vi "LargeNetworks.vi"() -> ()   [LabVIEW 2022 SP3]
uses:
  MOTION/TypeDefs/EL72xx_DMCOutputs.ctl
  MOTION/TypeDefs/EL72xx_DMCInputs.ctl
  SAFETY/TypeDefs/TwinSAFEGroupInfoData.ctl
  SAFETY/TypeDefs/FSLogicInputs.ctl
  SAFETY/TypeDefs/DeviceInfoData.ctl
  IO/TypeDefs/EL2008Outputs.ctl
  SAFETY/TypeDefs/TwinSAFETerminal.ctl
  <userlib>/Beckhoff-LabVIEW-Interface/Utilities/Notification/Buffered User-Event Data.ctl
  <userlib>/Beckhoff-LabVIEW-Interface/_DependsOn/Base/Read/Register E-Notification Buffered.vi
  <userlib>/Beckhoff-LabVIEW-Interface/_DependsOn/Base/Read/Read Sync.vi
  <userlib>/Beckhoff-LabVIEW-Interface/_DependsOn/Base/TypeResolver/Get TypeResolver.vi
  MOTION/Motion_Library.lvlib
  ADS/ADS_Library.lvlib
  SAFETY/Safety_Library.lvlib
  IO/IO_Library.lvlib
panel:
  out "bHasMatched 3":bool
  out "Write Status 3":bool
  in  "NI9472":T1
  in  "Digital Outputs 2":string="<PortInfo><Inputs><SymbolControlItems><SymbolControlItem GroupName=\"ADS Write\" GroupDescription=\"Parameters for ADS Write command\"><Parameters><Parameter Name=\"Name\">Box 17 (NI 9145).Module 1 (NI 9472).Digital Output.DO</Parameter><Parameter Name=\"SymbolName\">Box 17 (NI 9145).Module 1 (NI 9472).Digital Output.DO</Parameter><Parameter Name=\"SymbolType\">USINT</Parameter><Parameter Name=\"SymbolGuid\"></Parameter><Parameter Name=\"AmsNetId\">10.97.0.23.1.1</Parameter><Parameter Name=\"Port\">27911</Parameter><Parameter Name=\"IndexGroup\">#x0</Parameter><Parameter Name=\"IndexOffset\">#x0</Parameter><Parameter Name=\"BitSize\">8</Parameter><Parameter Name=\"CycleTime [ms]\">10</Parameter><Parameter Name=\"Timeout [ms]\">1000</Parameter></Parameters></SymbolControlItem></SymbolControlItems></Inputs><Outputs><SymbolControlItems /></Outputs></PortInfo>"
  out "error out 5":errorcluster
  in  "error in (no error) 2":errorcluster
  out "EL2904":T2
  out "EL1904":T2
  in  "stop":bool
  out "Read status? 3":bool
  out "RDataArray":variant[](array[variant])
  out "RData":variant
  out "Waveform Chart 2":dbl(graph)
  out "error out 4":errorcluster
  in  "error in 2":errorcluster
  in  "String":string="<PortInfo><Inputs><SymbolControlItems /></Inputs><Outputs><SymbolControlItems><SymbolControlItem GroupName=\"ADS Read\" GroupDescription=\"Parameters for ADS Read command\"><Parameters><Parameter Name=\"Name\">Term 15 (EL3255).AI Standard Channel 1.Value</Parameter><Parameter Name=\"SymbolName\">Term 15 (EL3255).AI Standard Channel 1.Value</Parameter><Parameter Name=\"SymbolType\">INT</Parameter><Parameter Name=\"SymbolGuid\"></Parameter><Parameter Name=\"AmsNetId\">10.97.0.23.1.1</Parameter><Parameter Name=\"Port\">27911</Parameter><Parameter Name=\"IndexGroup\">#x0</Parameter><Parameter Name=\"IndexOffset\">#x0</Parameter><Parameter Name=\"BitSize\">16</Parameter><Parameter Name=\"CycleTime [ms]\">10</Parameter><Parameter Name=\"Transmode\">3</Parameter><Parameter Name=\"Timeout [ms]\">1000</Parameter><Parameter Name=\"TCBufferSize [Samples]\">10</Parameter><Parameter Name=\"LVBufferSize [Samples]\">50</Parameter><Parameter Name=\"Expected min delay [ms]\">500</Parameter></Parameters></SymbolControlItem></SymbolControlItems></Outputs></PortInfo>"
  in  "Digital Outputs":string="<PortInfo><Inputs><SymbolControlItems><SymbolControlItem GroupName=\"ADS Write\" GroupDescription=\"Parameters for ADS Write command\"><Parameters><Parameter Name=\"Name\">Term 2 (EL2008).Channel 1.Output</Parameter><Parameter Name=\"SymbolName\">Term 2 (EL2008).Channel 1.Output</Parameter><Parameter Name=\"SymbolType\">BIT</Parameter><Parameter Name=\"SymbolGuid\"></Parameter><Parameter Name=\"AmsNetId\">10.97.0.23.1.1</Parameter><Parameter Name=\"Port\">27905</Parameter><Parameter Name=\"IndexGroup\">#x0</Parameter><Parameter Name=\"IndexOffset\">#x0</Parameter><Parameter Name=\"BitSize\">1</Parameter><Parameter Name=\"CycleTime [ms]\">2</Parameter><Parameter Name=\"Timeout [ms]\">1000</Parameter></Parameters></SymbolControlItem><SymbolControlItem GroupName=\"ADS Write\" GroupDescription=\"Parameters for ADS Write command\"><Parameters><Parameter Name=\"Name\">Term 2 (EL2008).Channel 2.Output</Parameter><Parameter Name=\"SymbolName\">Term 2 (EL2008).Channel 2.Output</Parameter><Parameter Name=\"SymbolType\">BIT</Parameter><Parameter Name=\"SymbolGuid\"></Parameter><Parameter Name=\"AmsNetId\">10.97.0.23.1.1</Parameter><Parameter Name=\"Port\">27905</Parameter><Parameter Name=\"IndexGroup\">#x0</Parameter><Parameter Name=\"IndexOffset\">#x0</Parameter><Parameter Name=\"BitSize\">1</Parameter><Parameter Name=\"CycleTime [ms]\">2</Parameter><Parameter Name=\"Timeout [ms]\">1000</Parameter></Parameters></SymbolControlItem><SymbolControlItem GroupName=\"ADS Write\" GroupDescription=\"Parameters for ADS Write command\"><Parameters><Parameter Name=\"Name\">Term 2 (EL2008).Channel 3.Output</Parameter><Parameter Name=\"SymbolName\">Term 2 (EL2008).Channel 3.Output</Parameter><Parameter Name=\"SymbolType\">BIT</Parameter><Parameter Name=\"SymbolGuid\"></Parameter><Parameter Name=\"AmsNetId\">10.97.0.23.1.1</Parameter><Parameter Name=\"Port\">27905</Parameter><Parameter Name=\"IndexGroup\">#x0</Parameter><Parameter Name=\"IndexOffset\">#x0</Parameter><Parameter Name=\"BitSize\">1</Parameter><Parameter Name=\"CycleTime [ms]\">2</Parameter><Parameter Name=\"Timeout [ms]\">1000</Parameter></Parameters></SymbolControlItem><SymbolControlItem GroupName=\"ADS Write\" GroupDescription=\"Parameters for ADS Write command\"><Parameters><Parameter Name=\"Name\">Term 2 (EL2008).Channel 4.Output</Parameter><Parameter Name=\"SymbolName\">Term 2 (EL2008).Channel 4.Output</Parameter><Parameter Name=\"SymbolType\">BIT</Parameter><Parameter Name=\"SymbolGuid\"></Parameter><Parameter Name=\"AmsNetId\">10.97.0.23.1.1</Parameter><Parameter Name=\"Port\">27905</Parameter><Parameter Name=\"IndexGroup\">#x0</Parameter><Parameter Name=\"IndexOffset\">#x0</Parameter><Parameter Name=\"BitSize\">1</Parameter><Parameter Name=\"CycleTime [ms]\">2</Parameter><Parameter Name=\"Timeout [ms]\">1000</Parameter></Parameters></SymbolControlItem><SymbolControlItem GroupName=\"ADS Write\" GroupDescription=\"Parameters for ADS Write command\"><Parameters><Parameter Name=\"Name\">Term 2 (EL2008).Channel 5.Output</Parameter><Parameter Name=\"SymbolName\">Term 2 (EL2008).Channel 5.Output</Parameter><Parameter Name=\"SymbolType\">BIT</Parameter><Parameter Name=\"SymbolGuid\"></Parameter><Parameter Name=\"AmsNetId\">10.97.0.23.1.1</Parameter><Parameter Name=\"Port\">27905</Parameter><Parameter Name=\"IndexGroup\">#x0</Parameter><Parameter Name=\"IndexOffset\">#x0</Parameter><Parameter Name=\"BitSize\">1</Parameter><Parameter Name=\"CycleTime [ms]\">2</Parameter><Parameter Name=\"Timeout [ms]\">1000</Parameter></Parameters></SymbolControlItem><SymbolControlItem GroupName=\"ADS Write\" GroupDescription=\"Parameters for ADS Write command\"><Parameters><Parameter Name=\"Name\">Term 2 (EL2008).Channel 6.Output</Parameter><Parameter Name=\"SymbolName\">Term 2 (EL2008).Channel 6.Output</Parameter><Parameter Name=\"SymbolType\">BIT</Parameter><Parameter Name=\"SymbolGuid\"></Parameter><Parameter Name=\"AmsNetId\">10.97.0.23.1.1</Parameter><Parameter Name=\"Port\">27905</Parameter><Parameter Name=\"IndexGroup\">#x0</Parameter><Parameter Name=\"IndexOffset\">#x0</Parameter><Parameter Name=\"BitSize\">1</Parameter><Parameter Name=\"CycleTime [ms]\">2</Parameter><Parameter Name=\"Timeout [ms]\">1000</Parameter></Parameters></SymbolControlItem><SymbolControlItem GroupName=\"ADS Write\" GroupDescription=\"Parameters for ADS Write command\"><Parameters><Parameter Name=\"Name\">Term 2 (EL2008).Channel 7.Output</Parameter><Parameter Name=\"SymbolName\">Term 2 (EL2008).Channel 7.Output</Parameter><Parameter Name=\"SymbolType\">BIT</Parameter><Parameter Name=\"SymbolGuid\"></Parameter><Parameter Name=\"AmsNetId\">10.97.0.23.1.1</Parameter><Parameter Name=\"Port\">27905</Parameter><Parameter Name=\"IndexGroup\">#x0</Parameter><Parameter Name=\"IndexOffset\">#x0</Parameter><Parameter Name=\"BitSize\">1</Parameter><Parameter Name=\"CycleTime [ms]\">2</Parameter><Parameter Name=\"Timeout [ms]\">1000</Parameter></Parameters></SymbolControlItem><SymbolControlItem GroupName=\"ADS Write\" GroupDescription=\"Parameters for ADS Write command\"><Parameters><Parameter Name=\"Name\">Term 2 (EL2008).Channel 8.Output</Parameter><Parameter Name=\"SymbolName\">Term 2 (EL2008).Channel 8.Output</Parameter><Parameter Name=\"SymbolType\">BIT</Parameter><Parameter Name=\"SymbolGuid\"></Parameter><Parameter Name=\"AmsNetId\">10.97.0.23.1.1</Parameter><Parameter Name=\"Port\">27905</Parameter><Parameter Name=\"IndexGroup\">#x0</Parameter><Parameter Name=\"IndexOffset\">#x0</Parameter><Parameter Name=\"BitSize\">1</Parameter><Parameter Name=\"CycleTime [ms]\">2</Parameter><Parameter Name=\"Timeout [ms]\">1000</Parameter></Parameters></SymbolControlItem></SymbolControlItems></Inputs><Outputs><SymbolControlItems /></Outputs></PortInfo>"
  out "error out 3":errorcluster
  out "Write Status 2":bool[](array[boolean])
  out "bHasMatched 2":bool[](array[boolean])
  in  "EL2008 Channels":T1
  in  "error in (no error)":errorcluster
  out "SymbolName":string
  in  "Start Notifications":bool=TRUE
  out "Waveform Chart":sgl(graph)
  in  "Stop Notifications":bool
  out "Has stopped?":bool
  out "Has started?":bool
  out "error out 2":errorcluster
  in  "error in":errorcluster
  in  "Counter":string="<PortInfo><Inputs><SymbolControlItems /></Inputs><Outputs><SymbolControlItems><SymbolControlItem GroupName=\"ADS Read\" GroupDescription=\"Parameters for ADS Read command\"><Parameters><Parameter Name=\"Name\">Term 14 (EL5021-0090).ENC Status.Counter value</Parameter><Parameter Name=\"SymbolName\">Term 14 (EL5021-0090).ENC Status.Counter value</Parameter><Parameter Name=\"SymbolType\">UDINT</Parameter><Parameter Name=\"SymbolGuid\"></Parameter><Parameter Name=\"AmsNetId\">10.97.0.23.1.1</Parameter><Parameter Name=\"Port\">27911</Parameter><Parameter Name=\"IndexGroup\">#x0</Parameter><Parameter Name=\"IndexOffset\">#x0</Parameter><Parameter Name=\"BitSize\">32</Parameter><Parameter Name=\"CycleTime [ms]\">10</Parameter><Parameter Name=\"Transmode\">3</Parameter><Parameter Name=\"Timeout [ms]\">1000</Parameter><Parameter Name=\"TCBufferSize [Samples]\">10</Parameter><Parameter Name=\"LVBufferSize [Samples]\">50</Parameter><Parameter Name=\"Expected min delay [ms]\">500</Parameter></Parameters></SymbolControlItem></SymbolControlItems></Outputs></PortInfo>"
  out "Read status? 2":bool[](array[boolean])
  out "error out":errorcluster
  out "output cluster 3":cluster{"SymbolName":string, "Cluster":T3} {"Cluster"."Project CRC" format="%x"}
  out "output cluster 4":cluster{"SymbolName":string, "FSLogic":T4}
  out "output cluster 5":T6
  in  "Safety Stop":bool
  in  "TwinSAFE":string="<PortInfo><Inputs><SymbolControlItems /></Inputs><Outputs><SymbolControlItems><SymbolControlItem GroupName=\"ADS Read\" GroupDescription=\"Parameters for ADS Read command\"><Parameters><Parameter Name=\"Name\">Term 13 (EL6910).Connection Info Data</Parameter><Parameter Name=\"SymbolName\">Term 13 (EL6910).Connection Info Data</Parameter><Parameter Name=\"SymbolType\">Connection Info Data_1_TYPE</Parameter><Parameter Name=\"SymbolGuid\"></Parameter><Parameter Name=\"AmsNetId\">10.97.0.23.1.1</Parameter><Parameter Name=\"Port\">27911</Parameter><Parameter Name=\"IndexGroup\">#x0</Parameter><Parameter Name=\"IndexOffset\">#x0</Parameter><Parameter Name=\"BitSize\">48</Parameter><Parameter Name=\"CycleTime [ms]\">10</Parameter><Parameter Name=\"Transmode\">3</Parameter><Parameter Name=\"Timeout [ms]\">1000</Parameter><Parameter Name=\"TCBufferSize [Samples]\">10</Parameter><Parameter Name=\"LVBufferSize [Samples]\">50</Parameter><Parameter Name=\"Expected min delay [ms]\">500</Parameter></Parameters></SymbolControlItem><SymbolControlItem GroupName=\"ADS Read\" GroupDescription=\"Parameters for ADS Read command\"><Parameters><Parameter Name=\"Name\">Term 13 (EL6910).Device Info Data</Parameter><Parameter Name=\"SymbolName\">Term 13 (EL6910).Device Info Data</Parameter><Parameter Name=\"SymbolType\">Device Info Data_1_TYPE</Parameter><Parameter Name=\"SymbolGuid\"></Parameter><Parameter Name=\"AmsNetId\">10.97.0.23.1.1</Parameter><Parameter Name=\"Port\">27911</Parameter><Parameter Name=\"IndexGroup\">#x0</Parameter><Parameter Name=\"IndexOffset\">#x0</Parameter><Parameter Name=\"BitSize\">48</Parameter><Parameter Name=\"CycleTime [ms]\">10</Parameter><Parameter Name=\"Transmode\">3</Parameter><Parameter Name=\"Timeout [ms]\">1000</Parameter><Parameter Name=\"TCBufferSize [Samples]\">10</Parameter><Parameter Name=\"LVBufferSize [Samples]\">50</Parameter><Parameter Name=\"Expected min delay [ms]\">500</Parameter></Parameters></SymbolControlItem><SymbolControlItem GroupName=\"ADS Read\" GroupDescription=\"Parameters for ADS Read command\"><Parameters><Parameter Name=\"Name\">Term 13 (EL6910).FSLOGIC Inputs</Parameter><Parameter Name=\"SymbolName\">Term 13 (EL6910).FSLOGIC Inputs</Parameter><Parameter Name=\"SymbolType\">FSLOGIC Inputs_1_TYPE</Parameter><Parameter Name=\"SymbolGuid\"></Parameter><Parameter Name=\"AmsNetId\">10.97.0.23.1.1</Parameter><Parameter Name=\"Port\">27911</Parameter><Parameter Name=\"IndexGroup\">#x0</Parameter><Parameter Name=\"IndexOffset\">#x0</Parameter><Parameter Name=\"BitSize\">16</Parameter><Parameter Name=\"CycleTime [ms]\">10</Parameter><Parameter Name=\"Transmode\">3</Parameter><Parameter Name=\"Timeout [ms]\">1000</Parameter><Parameter Name=\"TCBufferSize [Samples]\">10</Parameter><Parameter Name=\"LVBufferSize [Samples]\">50</Parameter><Parameter Name=\"Expected min delay [ms]\">500</Parameter></Parameters></SymbolControlItem><SymbolControlItem GroupName=\"ADS Read\" GroupDescription=\"Parameters for ADS Read command\"><Parameters><Parameter Name=\"Name\">Term 13 (EL6910).TwinSAFE Group Info Data.TwinSafeGroup1 Info Data</Parameter><Parameter Name=\"SymbolName\">Term 13 (EL6910).TwinSAFE Group Info Data.TwinSafeGroup1 Info Data</Parameter><Parameter Name=\"SymbolType\">INFODATA_GRP_3</Parameter><Parameter Name=\"SymbolGuid\"></Parameter><Parameter Name=\"AmsNetId\">10.97.0.23.1.1</Parameter><Parameter Name=\"Port\">27911</Parameter><Parameter Name=\"IndexGroup\">#x0</Parameter><Parameter Name=\"IndexOffset\">#x0</Parameter><Parameter Name=\"BitSize\">16</Parameter><Parameter Name=\"CycleTime [ms]\">10</Parameter><Parameter Name=\"Transmode\">3</Parameter><Parameter Name=\"Timeout [ms]\">1000</Parameter><Parameter Name=\"TCBufferSize [Samples]\">10</Parameter><Parameter Name=\"LVBufferSize [Samples]\">50</Parameter><Parameter Name=\"Expected min delay [ms]\">500</Parameter></Parameters></SymbolControlItem></SymbolControlItems></Outputs></PortInfo>"
  in  "Motion Stop":bool
  out "Read status?":bool
  out "data":T7
  in  "DMC Outputs":T8
  out "Write Status":bool
  out "bHasMatched":bool
  in  "Motion":string="<PortInfo><Inputs><SymbolControlItems><SymbolControlItem GroupName=\"ADS Write\" GroupDescription=\"Parameters for ADS Write command\"><Parameters><Parameter Name=\"Name\">Term 21 (EL7201-9014).DMC Outputs 32 Bit</Parameter><Parameter Name=\"SymbolName\">Term 21 (EL7201-9014).DMC Outputs 32 Bit</Parameter><Parameter Name=\"SymbolType\">DMC Outputs 32 Bit_1_TYPE</Parameter><Parameter Name=\"SymbolGuid\"></Parameter><Parameter Name=\"AmsNetId\">10.97.0.23.1.1</Parameter><Parameter Name=\"Port\">27911</Parameter><Parameter Name=\"IndexGroup\">#x0</Parameter><Parameter Name=\"IndexOffset\">#x0</Parameter><Parameter Name=\"BitSize\">320</Parameter><Parameter Name=\"CycleTime [ms]\">10</Parameter><Parameter Name=\"Timeout [ms]\">1000</Parameter></Parameters></SymbolControlItem></SymbolControlItems></Inputs><Outputs><SymbolControlItems><SymbolControlItem GroupName=\"ADS Read\" GroupDescription=\"Parameters for ADS Read command\"><Parameters><Parameter Name=\"Name\">Term 21 (EL7201-9014).DMC Inputs 32 Bit</Parameter><Parameter Name=\"SymbolName\">Term 21 (EL7201-9014).DMC Inputs 32 Bit</Parameter><Parameter Name=\"SymbolType\">DMC Inputs 32 Bit_1_TYPE</Parameter><Parameter Name=\"SymbolGuid\"></Parameter><Parameter Name=\"AmsNetId\">10.97.0.23.1.1</Parameter><Parameter Name=\"Port\">27911</Parameter><Parameter Name=\"IndexGroup\">#x0</Parameter><Parameter Name=\"IndexOffset\">#x0</Parameter><Parameter Name=\"BitSize\">512</Parameter><Parameter Name=\"CycleTime [ms]\">10</Parameter><Parameter Name=\"Transmode\">3</Parameter><Parameter Name=\"Timeout [ms]\">1000</Parameter><Parameter Name=\"TCBufferSize [Samples]\">10</Parameter><Parameter Name=\"LVBufferSize [Samples]\">50</Parameter><Parameter Name=\"Expected min delay [ms]\">500</Parameter></Parameters></SymbolControlItem></SymbolControlItems></Outputs></PortInfo>"
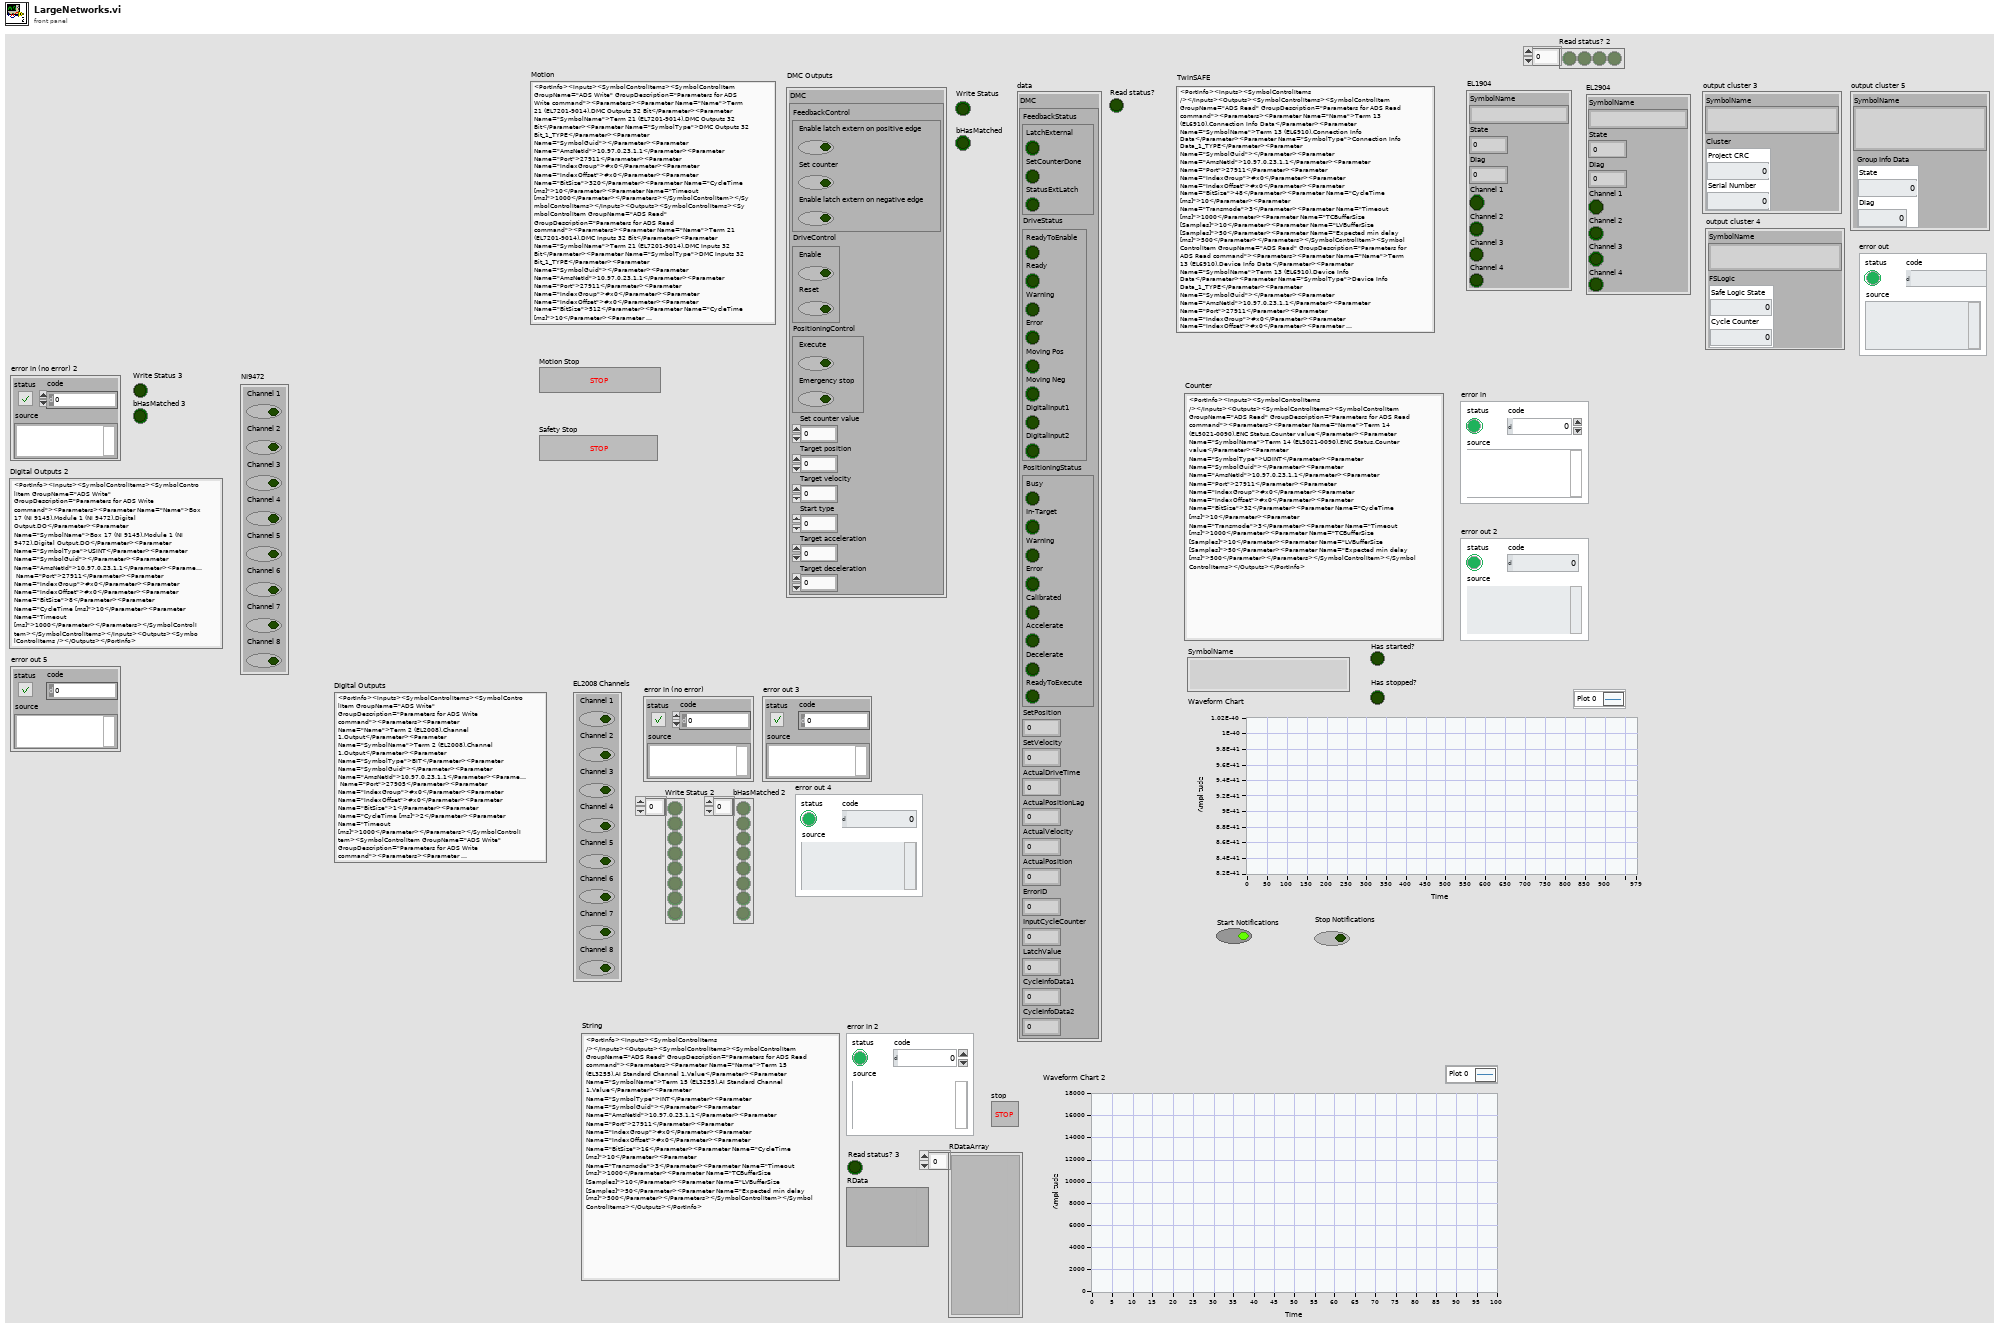
[diagram p1: front panel]
types:
  T1 = typedef "IO_Library.lvlib/EL2008Outputs.ctl" = cluster{"Channel 1":bool, "Channel 2":bool, "Channel 3":bool, "Channel 4":bool, "Channel 5":bool, "Channel 6":bool, "Channel 7":bool, "Channel 8":bool}
  T2 = typedef "TwinSAFETerminal.ctl" = cluster{"SymbolName":string, "State":dbl, "Diag":dbl, "Channel 1":bool, "Channel 2":bool, "Channel 3":bool, "Channel 4":bool}
  T3 = typedef "Safety_Library.lvlib/DeviceInfoData.ctl" = cluster{"Project CRC":u16, "Serial Number":u32}
  T4 = typedef "Safety_Library.lvlib/FSLogicInputs.ctl" = cluster{"Safe Logic State":u8, "Cycle Counter":u8}
  T5 = typedef "Safety_Library.lvlib/TwinSAFEGroupInfoData.ctl" = cluster{"State":u8, "Diag":u8}
  T6 = cluster{"SymbolName":string, "Group Info Data":T5}
  T7 = typedef "Motion_Library.lvlib/EL72xx_DMCInputs.ctl" = cluster{"DMC":cluster{"FeedbackStatus":cluster{"LatchExternal":bool, "SetCounterDone":bool, "StatusExtLatch":bool}, "DriveStatus":cluster{"ReadyToEnable":bool, "Ready":bool, "Warning":bool, "Error":bool, "Moving Pos":bool, "Moving Neg":bool, "DigitalInput1":bool, "DigitalInput2":bool}, "PositioningStatus":cluster{"Busy":bool, "In-Target":bool, "Warning":bool, "Error":bool, "Calibrated":bool, "Accelerate":bool, "Decelerate":bool, "ReadyToExecute":bool}, "SetPosition":dbl, "SetVelocity":dbl, "ActualDriveTime":dbl, "ActualPositionLag":dbl, "ActualVelocity":dbl, "ActualPosition":dbl, "ErrorID":dbl, "InputCycleCounter":dbl, "LatchValue":dbl, "CycleInfoData1":dbl, "CycleInfoData2":dbl}}
  T8 = typedef "Motion_Library.lvlib/EL72xx_DMCOutputs.ctl" = cluster{"DMC":cluster{"FeedbackControl":cluster{"Enable latch extern on positive edge":bool, "Set counter":bool, "Enable latch extern on negative edge":bool}, "DriveControl":cluster{"Enable":bool, "Reset":bool}, "PositioningControl":cluster{"Execute":bool, "Emergency stop":bool}, "Set counter value":i32, "Target position":i32, "Target velocity":i16, "Start type":u16, "Target acceleration":u16, "Target deceleration":u16}}
  T9 = typedef "Buffered User-Event Data.ctl" = cluster{"NotiHandle":u32, "Samples":i32, "BufferInfo":cluster{"Previous Overflow Samples":u32, "Missing Samples":u32, "Buffer Usage":dbl}, "RawData":u8[], "Timestamps":i64[]}
  T10 = cluster{"State":dbl, "State 2":dbl, "State 3":i8}
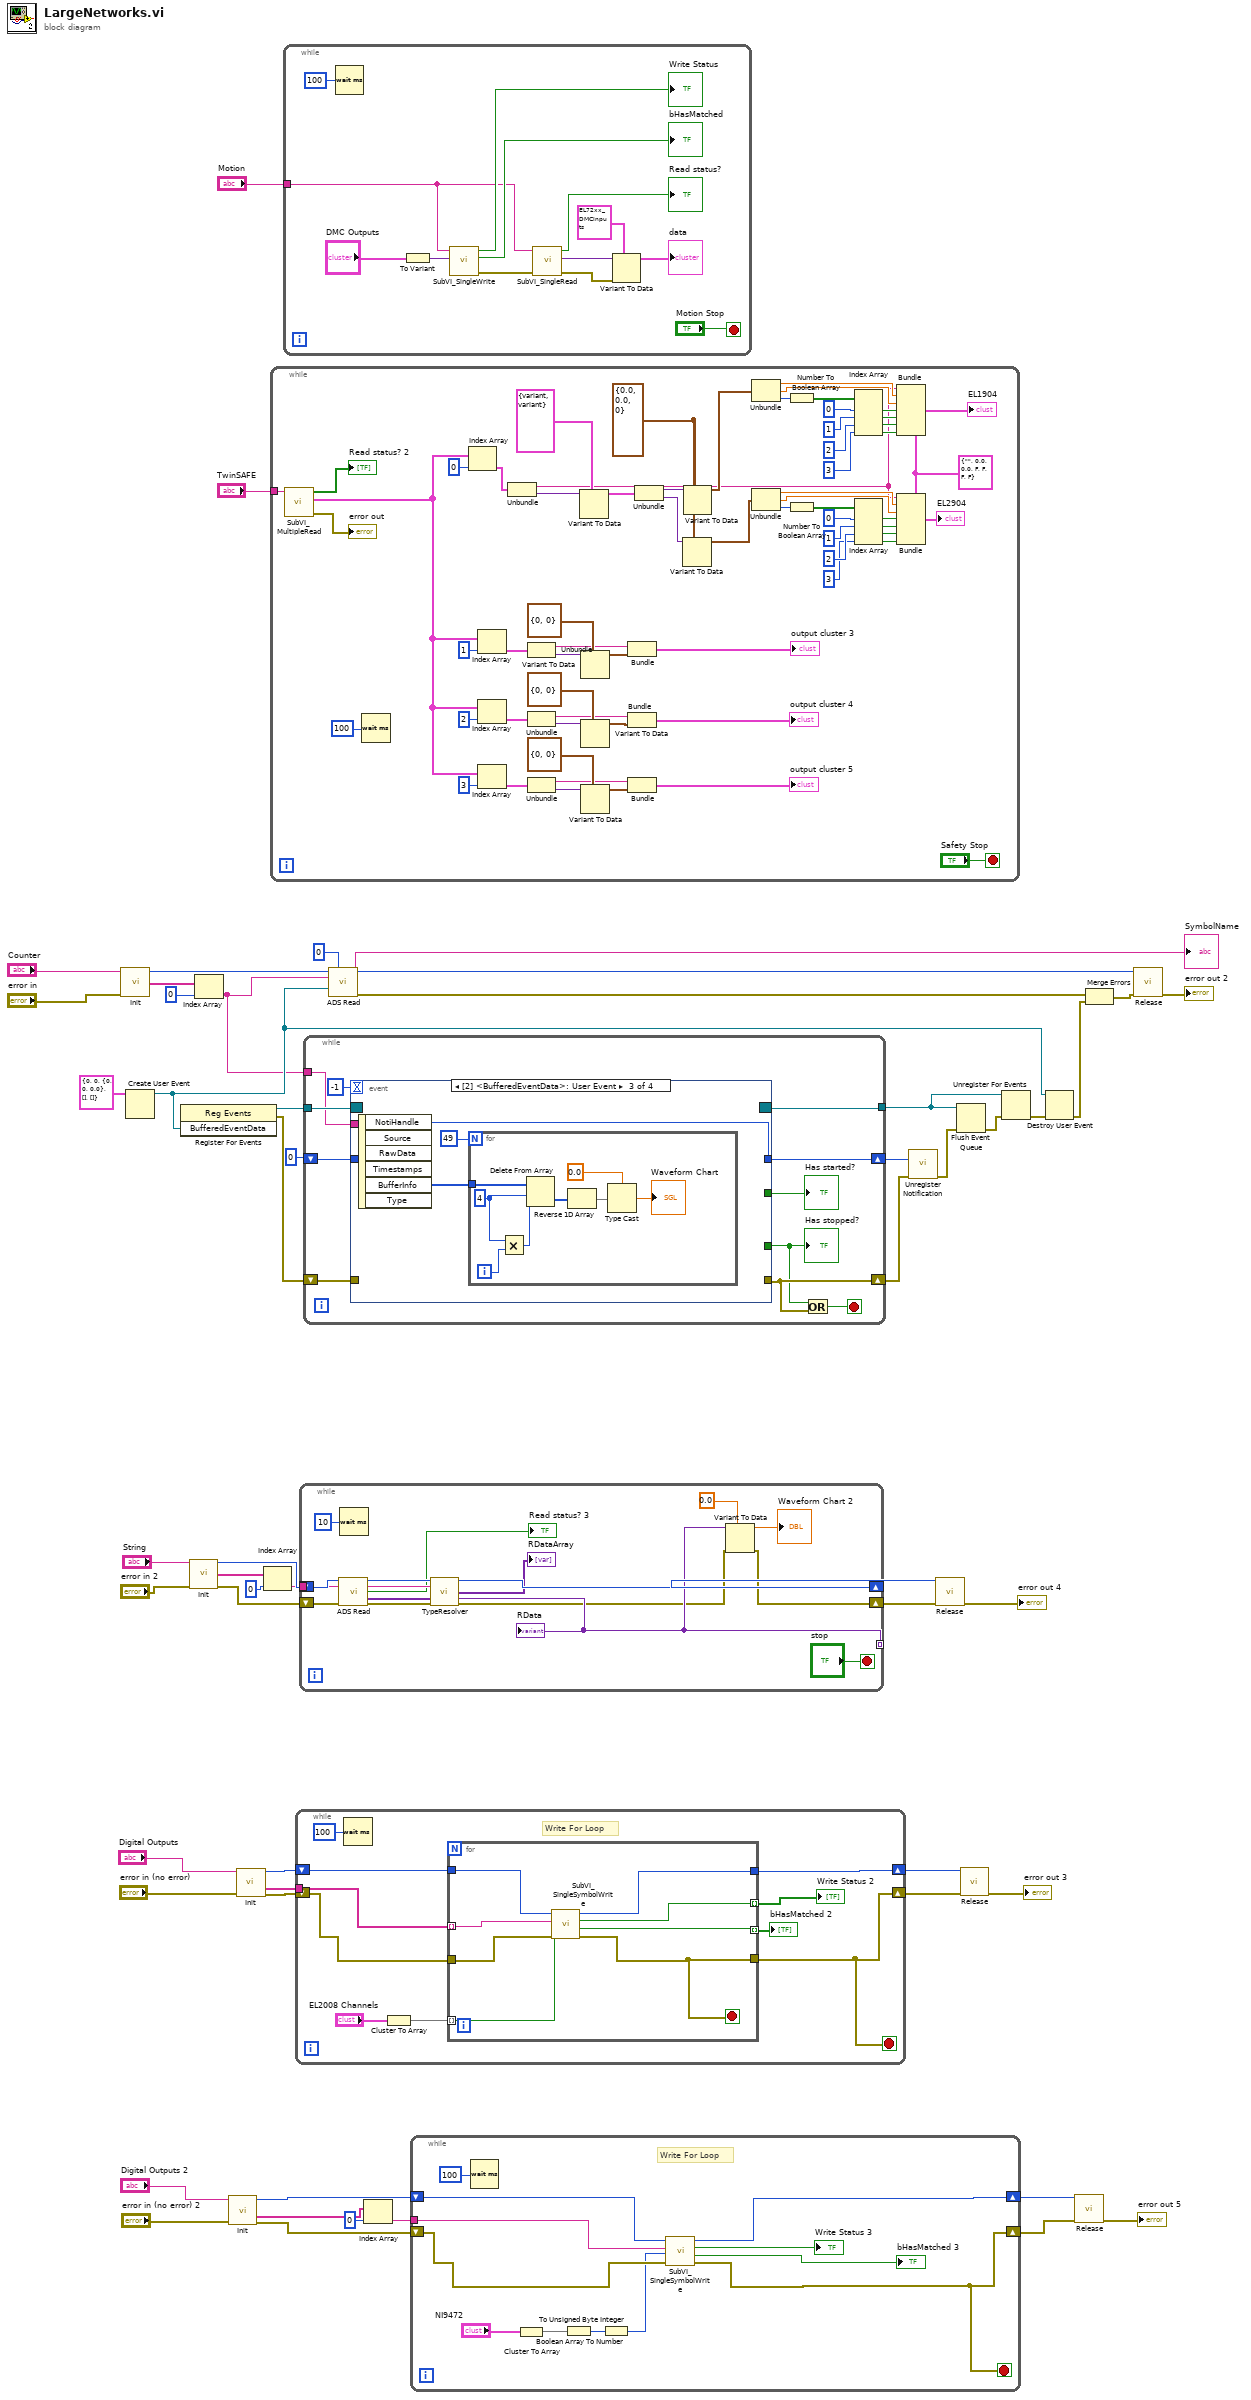
[diagram p0: block diagram]
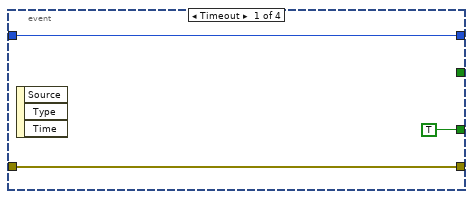
[diagram p2: hidden frame]
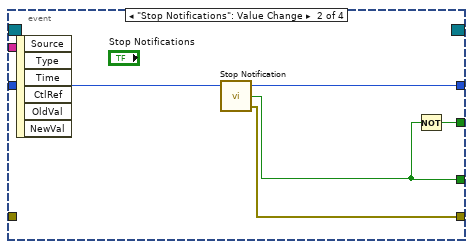
[diagram p3: hidden frame]
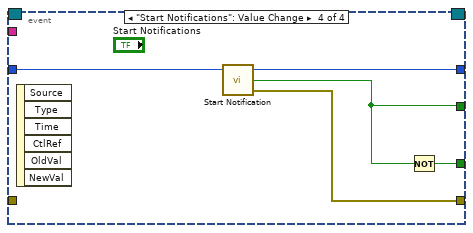
[diagram p4: hidden frame]
diagram:
  n1 = call <userlib>:"Init.vi"("XMLDescription"="Counter", "error in (no error)"="error in") -> ("Handle"=w31:u32, "ReadGrpSymbols"=w51:string[])  [unwired: 9 in, 3 out]
  n2 = Create User Event(user event datatype=T9 {"NotiHandle"=0, "Samples"=0, "BufferInfo"={"Previous Overflow Samples"=0, "Missing Samples"=0, "Buffer Usage"=0.0}, "RawData"=[], "Timestamps"=[]} ("BufferedEventData")) -> (user event=w40:refnum<user-event>)  [unwired: 1 in, 1 out]
  n3 = register-events(w40) -> (reference out=w45:refnum<event-registration>, error out=w35:errorcluster)  [unwired: 2 in]
  n4 = call <userlib>:"Init.vi"("XMLDescription"="String", "error in (no error)"="error in 2") -> ("Handle"=w18:u32, "ReadGrpSymbols"=w17:string[], "error out"=w19:errorcluster)  [unwired: 9 in, 2 out]
  n5 = Index Array(array=w51, index=0) -> (element=w32:string)
  n6 = call <userlib>:"Init.vi"("XMLDescription"="Digital Outputs 2", "error in (no error)"="error in (no error) 2") -> ("Handle"=w9:u32, "WriteGrpSymbols"=w3:string[], "error out"=w8:errorcluster)  [unwired: 9 in, 2 out]
  n7 = call <userlib>:"Init.vi"("XMLDescription"="Digital Outputs", "error in (no error)"="error in (no error)") -> ("Handle"=w26:u32, "WriteGrpSymbols"=w27:string[], "error out"=w25:errorcluster)  [unwired: 9 in, 2 out]
  n8 = Index Array(array=w17, index=0) -> (element=w15:string)
  n9 = while {
    tunnel: "TwinSAFE" -> [w119]
    stop <- "Safety Stop" stop-if-true
    w56 = T2 {"SymbolName"="", "State"=0.0, "Diag"=0.0, "Channel 1"=FALSE, "Channel 2"=FALSE, "Channel 3"=FALSE, "Channel 4"=FALSE} ("EL1904 2")
    w85 = T10 {"State"=0.0, "State 2"=0.0, "State 3"=0}
    n10 = call "SubVI_MultipleRead.vi"("String"=w119) -> ("error out"=→"error out":errorcluster, "Data"=w112:cluster{"SymbolName":string, "RData":variant}[], "Read status?"=→"Read status? 2":bool[])  [unwired: 8 in]
    n11 = Wait (ms)(milliseconds to wait=u32 100) -> ()  [unwired: 1 out]
    n12 = Index Array(array=w112, index=0) -> (element=w91:cluster{"SymbolName":string, "RData":variant})
    n13 = Index Array(array=w112, index=1) -> (element=w111:cluster{"SymbolName":string, "RData":variant})
    n14 = Index Array(array=w112, index=2) -> (element=w110:cluster{"SymbolName":string, "RData":variant})
    n15 = Index Array(array=w112, index=3) -> (element=w109:cluster{"SymbolName":string, "RData":variant})
    n16 = Unbundle(w91) -> ("SymbolName"=w58:string, "RData"=w90:variant)
    n17 = Unbundle(w111) -> ("SymbolName"=w102:string, "RData"=w106:variant)
    n18 = Unbundle(w110) -> ("SymbolName"=w101:string, "RData"=w107:variant)
    n19 = Unbundle(w109) -> ("SymbolName"=w100:string, "RData"=w108:variant)
    n20 = Variant To Data(type=cluster{variant, variant} {variant, variant}, Variant=w90) -> (data=w88:cluster{variant, variant})  [unwired: 1 in, 1 out]
    n21 = Variant To Data(type=T3 {"Project CRC"=0, "Serial Number"=0} ("Cluster"), Variant=w106) -> (data=w99:T3)  [unwired: 1 in, 1 out]
    n22 = Variant To Data(type=T4 {"Safe Logic State"=0, "Cycle Counter"=0} ("FSLogic"), Variant=w107) -> (data=w98:T4)  [unwired: 1 in, 1 out]
    n23 = Variant To Data(type=T5 {"State"=0, "Diag"=0} ("Group Info Data"), Variant=w108) -> (data=w97:T5)  [unwired: 1 in, 1 out]
    n24 = Bundle("SymbolName"=w102, "Cluster"=w99) -> (→"output cluster 3":cluster{"SymbolName":string, "Cluster":T3})  [unwired: 1 in]
    n25 = Bundle("SymbolName"=w101, "FSLogic"=w98) -> (→"output cluster 4":cluster{"SymbolName":string, "FSLogic":T4})  [unwired: 1 in]
    n26 = Bundle("SymbolName"=w100, "Group Info Data"=w97) -> (→"output cluster 5":T6)  [unwired: 1 in]
    n27 = Unbundle(w88) -> (w87:variant, w86:variant)
    n28 = Variant To Data(type=w85, Variant=w86) -> (data=w60:T10)  [unwired: 1 in, 1 out]
    n29 = Variant To Data(type=w85, Variant=w87) -> (data=w84:T10)  [unwired: 1 in, 1 out]
    n30 = Unbundle(w84) -> ("State"=w76:dbl, "State 2"=w77:dbl, "State 3"=w83:i8)
    n31 = Unbundle(w60) -> ("State"=w65:dbl, "State 2"=w66:dbl, "State 3"=w71:i8)
    n32 = Number To Boolean Array(number=w83) -> (Boolean array=w82:bool[])
    n33 = Number To Boolean Array(number=w71) -> (Boolean array=w70:bool[])
    n34 = Index Array(array=w82, index #1=0 ("index"), index #2=1 ("index"), index #3=2 ("index"), index #4=3 ("index")) -> (element #1=w75:bool, element #2=w74:bool, element #3=w73:bool, element #4=w72:bool)
    n35 = Index Array(array=w70, index #1=0 ("index"), index #2=1 ("index"), index #3=2 ("index"), index #4=3 ("index")) -> (element #1=w64:bool, element #2=w63:bool, element #3=w62:bool, element #4=w61:bool)
    n36 = Bundle(cluster=w56, "SymbolName"=w58, "State"=w76, "Diag"=w77, "Channel 1"=w75, "Channel 2"=w74, "Channel 3"=w73, "Channel 4"=w72) -> (→"EL1904":T2)
    n37 = Bundle(cluster=w56, "SymbolName"=w58, "State"=w65, "Diag"=w66, "Channel 1"=w64, "Channel 2"=w63, "Channel 3"=w62, "Channel 4"=w61) -> (→"EL2904":T2)
  }
  n38 = while {
    tunnel: "Motion" -> [w120]
    stop <- "Motion Stop" stop-if-true
    n39 = Wait (ms)(milliseconds to wait=u32 100) -> ()  [unwired: 1 out]
    n40 = To Variant(anything="DMC Outputs") -> (Variant=w124:variant)
    n41 = call "SubVI_SingleWrite.vi"("WData"=w124, "String"=w120) -> ("error out"=w123:errorcluster, "bHasMatched"=→"bHasMatched":bool, "Write Status"=→"Write Status":bool)  [unwired: 6 in, 1 out]
    n42 = call "SubVI_SingleRead.vi"("error in"=w123, "String"=w120) -> ("error out"=w129:errorcluster, "RData"=w130:variant, "Read status?"=→"Read status?":bool)  [unwired: 6 in]
    n43 = Variant To Data(error in=w129, type=T7 {"DMC"={"FeedbackStatus"={"LatchExternal"=FALSE, "SetCounterDone"=FALSE, "StatusExtLatch"=FALSE}, "DriveStatus"={"ReadyToEnable"=FALSE, "Ready"=FALSE, "Warning"=FALSE, "Error"=FALSE, "Moving Pos"=FALSE, "Moving Neg"=FALSE, "DigitalInput1"=FALSE, "DigitalInput2"=FALSE}, "PositioningStatus"={"Busy"=FALSE, "In-Target"=FALSE, "Warning"=FALSE, "Error"=FALSE, "Calibrated"=FALSE, "Accelerate"=FALSE, "Decelerate"=FALSE, "ReadyToExecute"=FALSE}, "SetPosition"=0.0, "SetVelocity"=0.0, "ActualDriveTime"=0.0, "ActualPositionLag"=0.0, "ActualVelocity"=0.0, "ActualPosition"=0.0, "ErrorID"=0.0, "InputCycleCounter"=0.0, "LatchValue"=0.0, "CycleInfoData1"=0.0, "CycleInfoData2"=0.0}} ("DMC Inputs"), Variant=w130) -> (data=→"data":T7)  [unwired: 1 out]
  }
  n44 = while {
    tunnel: w27 -> [w142]
    shift-right: [w137] -> w24
    shift-left: w26 -> [w139]
    shift-right: [w134] -> w23
    shift-left: w25 -> [w138]
    stop <- w134 stop-if-true
    # "Write For Loop"
    n45 = Wait (ms)(milliseconds to wait=u32 100) -> ()  [unwired: 1 out]
    n46 = Cluster To Array(cluster="EL2008 Channels") -> (array=w135:bool[])
    n47 = for {
      tunnel: w142 -> [w149] mode=indexing
      tunnel: w138 -> [w148]
      tunnel: w139 -> [w150]
      tunnel: [w144] -> w134
      tunnel: [w146] -> w140 mode=indexing
      tunnel: [w147] -> w141 mode=indexing
      tunnel: [w145] -> w137
      tunnel: w135 -> [w143] mode=indexing
      stop <- w144 stop-if-true
      n48 = call "SubVI_SingleSymbolWrite.vi"("error in"=w148, "WData"=w143, "SymbolName"=w149, "Handle In"=w150) -> ("error out"=w144:errorcluster, "bHasMatched"=w146:bool, "Write Status"=w147:bool, "Handle Out"=w145:u32)  [unwired: 4 in]
    }
    "bHasMatched 2" <- w140
    "Write Status 2" <- w141
  }
  n49 = while {
    tunnel: w15 -> [w165]
    shift-right: [w155] -> w14
    shift-left: w19 -> [w167]
    shift-right: [w160] -> w13
    shift-left: w18 -> [w166]
    tunnel: [w157] -> _ mode=indexing
    stop <- "stop" stop-if-true
    n50 = call-poly <userlib>:"ADS Read.vi"("Handle"=w166, "SymbolName"=w165, "error in (no error)"=w167) -> ("Handle"=w164:u32, "SymbolName"=w163:string, "Read status?"=→"Read status? 3":bool, "Ads Read Data"=w162:variant[], "error out"=w161:errorcluster)  [unwired: 8 in]
    n51 = Wait (ms)(milliseconds to wait=u32 10) -> ()  [unwired: 1 out]
    n52 = call-poly <userlib>:"TypeResolver.vi"("Handle"=w164, "SymbolName"=w163, "ADSRData"=w162, "error in"=w161) -> ("Handle"=w160:u32, "RDataArray"=→"RDataArray":variant[], "RData"=w157:variant, "error out"=w156:errorcluster)  [unwired: 8 in]
    "RData" <- w157
    n53 = Variant To Data(error in=w156, type=0.0, Variant=w157) -> (data=→"Waveform Chart 2":dbl, error out=w155:errorcluster)
  }
  n54 = while {
    tunnel: w45 -> [w177]
    shift-right: [w175] -> w33
    shift-left: u32 0 ("NotiHandle") -> [w176]
    tunnel: [w174] -> w41
    shift-right: [w172] -> w34
    shift-left: w35 -> [w173]
    tunnel: w32 -> [w170]
    stop <- w171 stop-if-true
    n55 = event shown="[2] <BufferedEventData>: User Event" {
      selector: w177 -> [_ _ _ _]
      dyn-events: [_ _ _ _] -> w174
      timeout: -1 -> [_ _ _ _]
      tunnel: w176 -> [w181 w186 _ w201]
      tunnel: [w181 w185 w189 w202] -> w175
      tunnel: [TRUE ("Has stopped?") w182 _ w199] -> w168
      tunnel: w173 -> [w180 _ _ _]
      tunnel: [w180 w184 _ w200] -> w172
      tunnel: w170 -> [_ _ _ _]
      tunnel: [_ w183 _ w198] -> w169
      event Timeout {
        n56 = event-data() -> ()  [unwired: 1 in, 3 out]
      }
      event "Stop Notifications": Value Change {
        n57 = event-data() -> ()  [unwired: 1 in, 6 out]
        n58 = call <userlib>:"Stop Notification.vi"("Reader Handle"=w186) -> ("error out"=w184:errorcluster, "Has stopped?"=w182:bool, "Reader Handle"=w185:u32)  [unwired: 2 in]
        n59 = Not(x=w182) -> (.not. x?=w183:bool)
      }
      event User Event {
        n60 = event-data() -> ("NotiHandle"=w189:u32, "RawData"=w187:u8[])  [unwired: 1 in, 4 out]
        n61 = for {
          N: 49 -> [_]
          tunnel: w187 -> [w197]
          i -> [w196]
          w190 = 4 ("length")
          n62 = Multiply(x=w190, y=w196) -> (x*y=w195:i32)
          n63 = Delete From Array(array=w197, length=w190, index=w195) -> (deleted portion=w191:u8[])  [unwired: 1 out]
          n64 = Reverse 1D Array(array=w191) -> (reversed array=w194:u8[])
          n65 = Type Cast(type=sgl 0.0, x=w194) -> (*(type *) &x=→"Waveform Chart":sgl)
        }
      }
      event "Start Notifications": Value Change {
        n66 = event-data() -> ()  [unwired: 1 in, 6 out]
        n67 = call <userlib>:"Start Notification.vi"("Reader Handle"=w201) -> ("error out"=w200:errorcluster, "Has started?"=w198:bool, "Reader Handle"=w202:u32)  [unwired: 2 in]
        n68 = Not(x=w198) -> (.not. x?=w199:bool)
      }
    }
    "Has stopped?" <- w168
    "Has started?" <- w169
    n69 = Or(x=w168, y=w172) -> (x .or. y?=w171:bool)
  }
  n70 = call-poly <userlib>:"ADS Read.vi"("Handle"=w31, "ElapseTimeMs"=u64 0, "SymbolName"=w32, "Noti. E-Buffered Event Ref"=w40) -> ("Handle"=w37:u32, "SymbolName"=→"SymbolName":string, "error out"=w39:errorcluster)  [unwired: 9 in]
  n71 = Index Array(array=w3, index=0) -> (element=w1:string)
  n72 = while {
    shift-right: [w212] -> w7
    shift-left: w9 -> [w214]
    shift-right: [w211] -> w6
    shift-left: w8 -> [w213]
    tunnel: w1 -> [w204]
    stop <- w211 stop-if-true
    # "Write For Loop"
    n73 = Wait (ms)(milliseconds to wait=u32 100) -> ()  [unwired: 1 out]
    n74 = Cluster To Array(cluster="NI9472") -> (array=w209:bool[])
    n75 = Boolean Array To Number(Boolean array=w209) -> (number=w208:u32)
    n76 = To Unsigned Byte Integer(number=w208) -> (unsigned 8bit integer=w207:u8)
    n77 = call "SubVI_SingleSymbolWrite.vi"("error in"=w213, "WData"=w207, "SymbolName"=w204, "Handle In"=w214) -> ("error out"=w211:errorcluster, "bHasMatched"=→"bHasMatched 3":bool, "Write Status"=→"Write Status 3":bool, "Handle Out"=w212:u32)  [unwired: 4 in]
  }
  n78 = call <userlib>:"Unregister Notification.vi"("Reader Handle"=w33, "error in"=w34) -> ("error out"=w36:errorcluster)  [unwired: 10 in, 3 out]
  n79 = call <userlib>:"Release.vi"("Handle"=w13, "error in (no error)"=w14) -> ("error out"=→"error out 4":errorcluster)  [unwired: 13 in]
  n80 = Flush Event Queue(0:w41, 3:w36) -> (11:w42:errorcluster)  [unwired: 4 in, 2 out]
  n81 = call <userlib>:"Release.vi"("Handle"=w24, "error in (no error)"=w23) -> ("error out"=→"error out 3":errorcluster)  [unwired: 13 in]
  n82 = Unregister For Events(event registration refnum=w41, error in=w42) -> (error out=w43:errorcluster)
  n83 = Destroy User Event(user event=w40, error in=w43) -> (error out=w38:errorcluster)
  n84 = call <userlib>:"Release.vi"("Handle"=w7, "error in (no error)"=w6) -> ("error out"=→"error out 5":errorcluster)  [unwired: 13 in]
  n85 = Merge Errors(w39, w38) -> (w47:errorcluster)
  n86 = call <userlib>:"Release.vi"("Handle"=w37, "error in (no error)"=w47) -> ("error out"=→"error out 2":errorcluster)  [unwired: 13 in]
